vi "Periodic Tasks.vi"(8 "error in":errorcluster) -> ()   [LabVIEW 2013]
doc: "This VI runs in parallel to other tasks. It can contain as many user-defined periodic loops as you need. These can carry out PID or other sorts of timed response."
uses:
  <vilib>/Rock Robotics/SystemInterfaces/Utilities/FPGA_UtilitiesLED Source.ctl
  <vilib>/Rock Robotics/SystemInterfaces/Utilities/FPGA_UtilitiesLED State.ctl
  Robot Global Data.vi
  Global.vi
  <vilib>/addons/control/pid/NI_PID_pid.lvlib
  <vilib>/addons/control/pid/pid.llb/PID Control Input Filter (DBL).vi
panel:
  in  "stop":bool
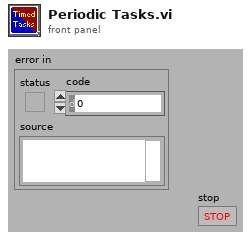
[diagram p1: front panel]
types:
  T1 = typedef "WPI_EncoderDevRef.ctl" = cluster{"DevStatus":errorcluster, "EncoderIndex":T2, "CounterIndex":T3, "DistancePerCount":dbl, "Decoding Type":T4}
  T2 = typedef "FPGA_EncoderIdx.ctl" = enum8{"Enc 0", "Enc 1", "Enc 2", "Enc 3", "Invalid"}
  T3 = typedef "FPGA_CounterCtrSystemIndex.ctl" = enum8{"Ctr 0", "Ctr 1", "Ctr 2", "Ctr 3", "Ctr 4", "Ctr 5", "Ctr 6", "Ctr 7", "Invalid"}
  T4 = typedef "WPI_EncoderType.ctl" = enum16{"1x", "2x", "4x"}
  T5 = typedef "FPGA_UtilitiesLED State.ctl" = enum16{"Off", "On", "Toggle"}
  T6 = typedef "FPGA_UtilitiesLED Source.ctl" = enum16{"User LED", "FPGA LED"}
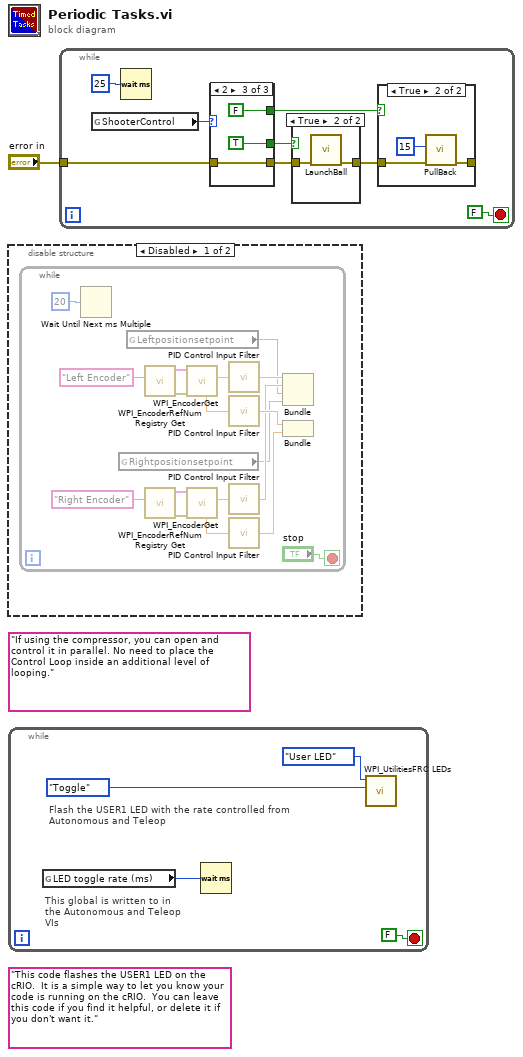
[diagram p0: block diagram]
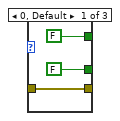
[diagram p4: hidden frame]
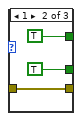
[diagram p5: hidden frame]
diagram:
  (unwired) "If using the compressor, you can open and control it in parallel. No need to place the Control Loop inside an additional level of looping."
  (unwired) "This code flashes the USER1 LED on the cRIO.  It is a simple way to let you know your code is running on the cRIO.  You can leave this code if you find it helpful, or delete it if you don't want it."
  n1 = disable-structure shown="Disabled" {
    frame Disabled {
      n2 = while {
        stop <- "stop" stop-if-true
        n3 = Wait Until Next ms Multiple(millisecond multiple=u32 20) -> ()  [unwired: 1 out]
        n4 = global read "Global.vi" "Rightpositionsetpoint"() -> (w3)
        n5 = global read "Global.vi" "Leftpositionsetpoint"() -> (w2)
        n6 = call <vilib>:"WPI_EncoderRefNum Registry Get.vi"("refnum name"="Left Encoder") -> ("error out"=w16:errorcluster, "EncoderDevRef"=w15:T1)  [unwired: 9 in]
        n7 = call <vilib>:"WPI_EncoderRefNum Registry Get.vi"("refnum name"="Right Encoder") -> ("error out"=w14:errorcluster, "EncoderDevRef"=w13:T1)  [unwired: 9 in]
        n8 = call <vilib>:"WPI_EncoderGet.vi"("error in (no error)"=w16, "EncoderDevRef"=w15) -> ("Distance"=w7:dbl, "Rate"=w11:dbl)  [unwired: 4 in, 4 out]
        n9 = call <vilib>:"WPI_EncoderGet.vi"("error in (no error)"=w14, "EncoderDevRef"=w13) -> ("Distance"=w6:dbl, "Rate"=w10:dbl)  [unwired: 4 in, 4 out]
        n10 = call-poly <vilib>:"PID Control Input Filter.vi"("input"=w7) -> ("output"=w5:dbl)  [unwired: 4 in]
        n11 = call-poly <vilib>:"PID Control Input Filter.vi"("input"=w11) -> ("output"=w9:dbl)  [unwired: 4 in]
        n12 = call-poly <vilib>:"PID Control Input Filter.vi"("input"=w6) -> ("output"=w4:dbl)  [unwired: 4 in]
        n13 = call-poly <vilib>:"PID Control Input Filter.vi"("input"=w10) -> ("output"=w8:dbl)  [unwired: 4 in]
        n14 = Bundle("output"=w5, "output"=w4, "Leftpositionsetpoint"=w2, "Rightpositionsetpoint"=w3) -> ()  [unwired: 1 in, 1 out]
        n15 = Bundle("output"=w9, "output"=w8) -> ()  [unwired: 1 in, 1 out]
      }
    }
    frame Enabled {
    }
  }
  n16 = while {
    stop <- FALSE stop-if-true
    # "This global is written to in the Autonomous and Teleop VIs"
    # "Flash the USER1 LED with the rate controlled from Autonomous and Teleop"
    n17 = global read "Robot Global Data.vi" "LED toggle rate (ms)"() -> (w20:u32)
    n18 = Wait (ms)(milliseconds to wait=w20) -> ()  [unwired: 1 out]
    n19 = call <vilib>:"WPI_UtilitiesFRC LEDs.vi"("State"=FPGA_UtilitiesLED_State."Toggle", "LED Type"=FPGA_UtilitiesLED_Source."User LED") -> ()  [unwired: 1 in, 9 out]
  }
  n20 = while {
    tunnel: "error in" -> [w28]
    stop <- FALSE stop-if-true
    n21 = global read "Robot Global Data.vi" "ShooterControl"() -> (w24:u32)
    n22 = Wait (ms)(milliseconds to wait=u32 25) -> ()  [unwired: 1 out]
    n23 = case shown="2" w24 {
      tunnel: w28 -> [w39 w42 w45]
      tunnel: [w39 w42 w45] -> w25
      tunnel: [FALSE TRUE TRUE] -> w29
      tunnel: [FALSE TRUE FALSE] -> w27
      frame 0, Default {
      }
      frame 1 {
      }
      frame 2 {
      }
    }
    n24 = case shown="True" w29 {
      tunnel: w25 -> [w36 w38]
      tunnel: [w36 w37] -> w26
      frame False {
      }
      frame True {
        n25 = call "LaunchBall.vi"("error in (no error)"=w38) -> ("error out"=w37:errorcluster)  [unwired: 10 in]
      }
    }
    n26 = case shown="True" w27 {
      tunnel: w26 -> [w32 w35]
      tunnel: [w32 w34] -> _
      frame False {
      }
      frame True {
        n27 = call "PullBack.vi"("error in (no error)"=w35, "Timeout (s)"=15) -> ("error out"=w34:errorcluster)  [unwired: 9 in]
      }
    }
  }
